vi "Build Tree.vi"(5 "Defer Updates (T)":bool=TRUE, 7 "Tree":refnum<vi>, 8 "error in (no error)":errorcluster, 11 "Tree Map in":refnum<class "Tree Map.lvclass">) -> (0 "error out":errorcluster, 3 "Tree Map out":refnum<class "Tree Map.lvclass">)   [LabVIEW 2023, in "VI Properties Editor.lvlib" / "Tree Map.lvlib" / "Tree Map.lvclass"]
uses:
  Tree Map.lvclass
  Tree Map.lvclass/Tree Map.ctl
  Tree Map.lvlib
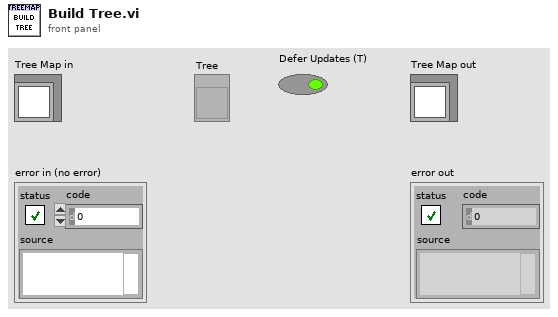
[diagram p1: front panel]
types:
  T1 = typedef "VI Properties Editor.lvlib/Tree Map.lvlib/Tree Map.lvclass/Tree Entry.ctl" = cluster{"Hierarchy":string[], "Name":string, "Columns":string[], "BG Color":u32, "Leaf":bool, "Symbol":string}
  T2 = typedef "imagedata.ctl" = cluster{"image type":i32, "image depth":i32, "image":u8[], "mask":u8[], "colors":u32[], "Rectangle":cluster{"left":i16, "top":i16, "right":i16, "bottom":i16}}
  T3 = map{string, cluster{"index":i32, "image data":T2}}
  T4 = typedef "LVNodeAndColumnTypeDef.ctl" = cluster{"Node":string, "Column":i32}
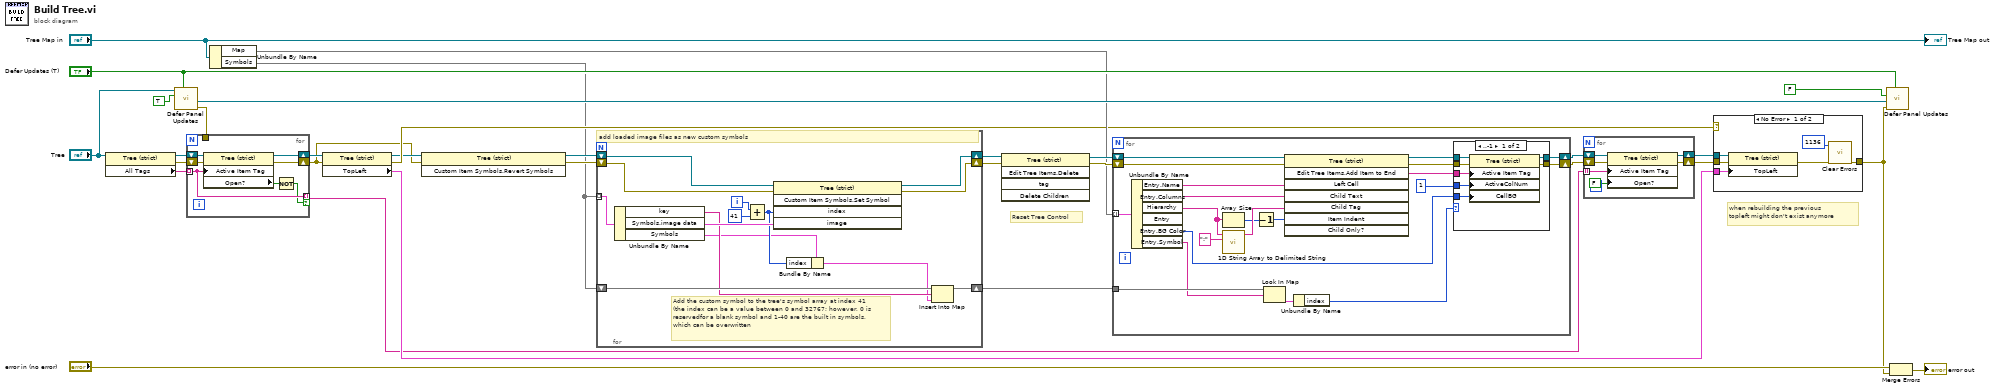
[diagram p0: block diagram]
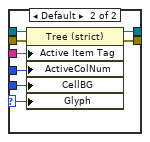
[diagram p3: hidden frame]
diagram:
  # "when rebuilding the previous\ntopleft might don't exist anymore"
  # "Reset Tree Control"
  n1 = property class="Tree (strict)"(reference="Tree") -> (reference out=w27:refnum<vi>, error out=w14:errorcluster, "All Tags"=w28:string[])  [unwired: 1 in]
  n2 = call "Defer Panel Updates.vi"("Set Defer (T)"="Defer Updates (T)", "Defer"=TRUE, "Tree (Front Panel)"="Tree") -> ("error out"=w15:errorcluster, "Front Panel"=w19:refnum<vi>)  [unwired: 7 in]
  n3 = for {
    tunnel: w28 -> [w37] mode=indexing
    shift-right: [w35] -> w26
    shift-left: w27 -> [w39]
    tunnel: [w37] -> w25 mode=indexing if=w36
    tunnel: w15 -> [_]
    shift-right: [w33] -> w5
    shift-left: w14 -> [w34]
    n4 = property class="Tree (strict)"(reference=w39, error in=w34, "Active Item Tag"=w37) -> (reference out=w35:refnum<vi>, error out=w33:errorcluster, "Open?"=w38:bool)
    n5 = Not(x=w38) -> (.not. x?=w36:bool)
  }
  n6 = Unbundle By Name("Tree Map in") -> ("Map"=w16:map{string[], T1}, "Symbols"=w3:T3)
  n7 = property class="Tree (strict)"(reference=w26, error in=w5) -> (reference out=w8:refnum<vi>, error out=w9:errorcluster, "TopLeft"=w29:T4)
  n8 = invoke on="Invoke Node" class="Tree (strict)" method="Custom Item Symbols.Revert Symbols"(reference=w8, error in=w5) -> (reference out=w7:refnum<vi>, error out=w6:errorcluster)  [unwired: 1 in, 1 out]
  n9 = for {
    shift-right: [w51] -> w1
    shift-left: w7 -> [w53]
    shift-right: [w50] -> w4
    shift-left: w6 -> [w52]
    tunnel: w3 -> [w46] mode=indexing
    shift-right: [w42] -> w2
    shift-left: w3 -> [w44]
    i -> [w49]
    # "Add the custom symbol to the tree's symbol array at index 41 (the index can be a value between 0 and 32767; however, 0 is reservedfor a blank symbol and 1-40 are the built in symbols, which can be overwritten"
    # "add loaded image files as new custom symbols"
    n10 = Unbundle By Name(w46) -> ("key"=w43:string, "Symbols.image data"=w48:T2, "Symbols"=w40:cluster{"index":i32, "image data":T2})
    n11 = Add(x=w49, y=41 ("Index")) -> (x+y=w45:i32)
    n12 = invoke on="Invoke Node" class="Tree (strict)" method="Custom Item Symbols.Set Symbol"(reference=w53, error in=w52, "index"=w45, "image"=w48) -> (reference out=w51:refnum<vi>, error out=w50:errorcluster)  [unwired: 1 in, 3 out]
    n13 = Bundle By Name(cluster=w40, "index"=w45) -> (w41:cluster{"index":i32, "image data":T2})
    n14 = Insert Into Map(map in=w44, key=w43, value=w41) -> (map out=w42:T3)  [unwired: 2 out]
  }
  n15 = invoke class="Tree (strict)" method="Edit Tree Items.Delete"(reference=w1, error in=w4) -> (reference out=w30:refnum<vi>, error out=w32:errorcluster)  [unwired: 3 in, 3 out]
  n16 = for {
    shift-right: [w60] -> w23
    shift-left: w30 -> [w74]
    tunnel: w16 -> [w65] mode=indexing
    shift-right: [w59] -> w13
    shift-left: w32 -> [w67]
    tunnel: w2 -> [w58]
    n17 = Unbundle By Name(w65) -> ("Entry.Name"=w68:string, "Entry.Columns"=w69:string[], "Hierarchy"=w66:string[], "Entry.BG Color"=w54:u32, "Entry.Symbol"=w55:string)  [unwired: 1 out]
    n18 = Array Size(array=w66) -> (size(s)=w71:i32)
    n19 = call <vilib>:"1D String Array to Delimited String.vi"("delimiter"=":", "string array"=w66) -> ("delimited string"=w72:string)  [unwired: 9 in]
    n20 = Decrement(x=w71) -> (x-1=w70:i32)
    n21 = Look In Map(map=w58, key=w55) -> (value=w57:cluster{"index":i32, "image data":T2})  [unwired: 1 in, 1 out]
    n22 = invoke class="Tree (strict)" method="Edit Tree Items.Add Item to End"(reference=w74, error in=w67, "Left Cell"=w68, "Child Text"=w69, "Child Tag"=w72, "Item Indent"=w70) -> (reference out=w64:refnum<vi>, error out=w63:errorcluster, "Edit Tree Items:Add Item to End"=w62:string)  [unwired: 2 in, 5 out]
    n23 = Unbundle By Name(w57) -> ("index"=w56:i32)
    n24 = case shown="..-1" w56 {
      selector: w56 -> [_ w82]
      tunnel: w64 -> [w80 w89]
      tunnel: w63 -> [w81 w88]
      tunnel: w62 -> [w75 w87]
      tunnel: 1 ("Active Cell:Active Column Number") -> [w76 w86]
      tunnel: [w78 w85] -> w60
      tunnel: [w79 w84] -> w59
      tunnel: w54 -> [w77 w83]
      frame ..-1 {
        n25 = property class="Tree (strict)"(reference=w80, error in=w81, "Active Item Tag"=w75, "ActiveColNum"=w76, "CellBG"=w77) -> (reference out=w78:refnum<vi>, error out=w79:errorcluster)
      }
      frame Default {
        n26 = property class="Tree (strict)"(reference=w89, error in=w88, "Active Item Tag"=w87, "ActiveColNum"=w86, "CellBG"=w83, "Glyph"=w82) -> (reference out=w85:refnum<vi>, error out=w84:errorcluster)
      }
    }
  }
  n27 = for {
    shift-right: [w94] -> w24
    shift-left: w23 -> [w95]
    tunnel: w25 -> [w92] mode=indexing
    shift-right: [w90] -> w12
    shift-left: w13 -> [w91]
    n28 = property class="Tree (strict)"(reference=w95, error in=w91, "Active Item Tag"=w92, "Open?"=FALSE ("Active Item:Open?")) -> (reference out=w94:refnum<vi>, error out=w90:errorcluster)
  }
  n29 = case shown="No Error" w9 {
    tunnel: w29 -> [w101 _]
    tunnel: w24 -> [w100 _]
    tunnel: w12 -> [w99 w102]
    tunnel: [w97 w102] -> w10
    frame No Error {
      n30 = property class="Tree (strict)"(reference=w100, error in=w99, "TopLeft"=w101) -> (error out=w98:errorcluster)  [unwired: 1 out]
      n31 = call <vilib>:"Clear Errors.vi"("error in (no error)"=w98, "specific error code to clear (0: all)"=1136) -> ("error out"=w97:errorcluster)  [unwired: 4 in, 1 out]
    }
    frame Error {
    }
  }
  n32 = call "Defer Panel Updates.vi"("Set Defer (T)"="Defer Updates (T)", "error in (no error)"=w10, "Front Panel (Lookup)"=w19, "Defer"=FALSE ("Defer Panel Updates")) -> ()  [unwired: 6 in, 2 out]
  n33 = Merge Errors("error in (no error)", w10) -> (→"error out":errorcluster)
  "Tree Map out" <- "Tree Map in"
